vi "get_config_cluster.vi"(8 "error in (no error)":errorcluster, 11 "GenericPlugin in":refnum<class "DetectorYK090623DAQmxAnalog.lvclass">) -> (0 "error out":errorcluster, 2 "config cluster (variant)":variant, 3 "GenericPlugin out":refnum<class "DetectorYK090623DAQmxAnalog.lvclass">)   [LabVIEW 2010, in "DetectorYK090623DAQmxAnalog.lvclass"]
uses:
  DetectorYK090623DAQmxAnalog.lvclass
  DetectorYK090623DAQmxAnalog.lvclass/DetectorYK090623DAQmxAnalog.ctl
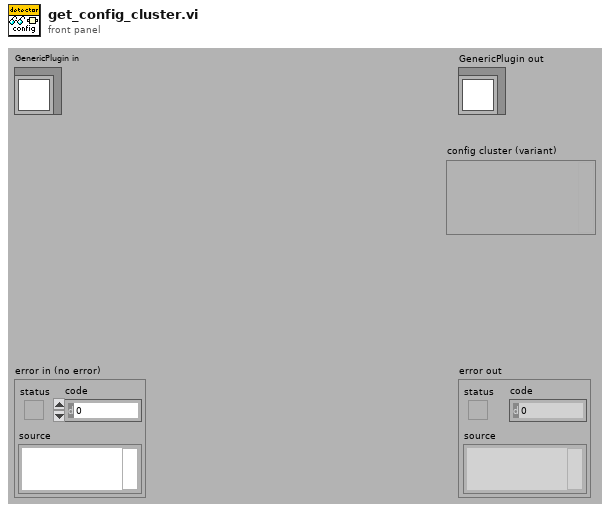
[diagram p1: front panel]
types:
  T1 = typedef "DetectorYK090623DAQmxAnalog.lvclass/config_data_cluster.ctl" = cluster{"manufacturer specification":T2, "type":T3, "LSID":T4, "default voltage":dbl[unit], "analog out":T5}
  T2 = typedef "GenericComponent.lvclass/manufacturer_specification_cluster.ctl" = cluster{"manufacturer":string, "model":string, "serial number":string, "lot number":string}
  T3 = typedef "GenericDetector.lvclass/type_enum.ctl" = enum16{"CCD", "IntensifiedCCD", "AnalogVideo", "PMT", "Photodiode", "Spectoscropy", "LifetimeImaging", "CorrelationSpectroscopy", "FTIR", "EM-CCD", "APD", "CMOS", "Unknown"}
  T4 = typedef "LSID_cluster.ctl" = cluster{"identifier":string, "revision":i32}
  T5 = typedef "plugin_specification.ctl" = cluster{"class path":string, "configuration":string, "label":string, "settings name":string}
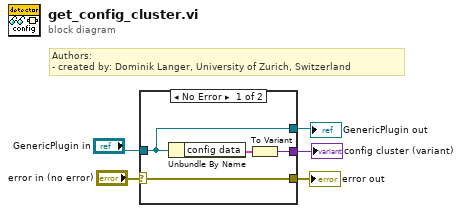
[diagram p0: block diagram]
diagram:
  # "Authors: \n- created by: Dominik Langer, University of Zurich, Switzerland"
  n1 = case shown="No Error" "error in (no error)" {
    selector: "error in (no error)" -> [w7 w11]
    tunnel: "GenericPlugin in" -> [w6 w10]
    tunnel: [w8 _] -> w2
    tunnel: [w7 w11] -> w3
    tunnel: [w6 w10] -> w1
    frame No Error {
      n2 = Unbundle By Name(w6) -> ("config data"=w9:T1)
      n3 = To Variant(anything=w9) -> (Variant=w8:variant)
    }
    frame Error {
    }
  }
  "error out" <- w3
  "GenericPlugin out" <- w1
  "config cluster (variant)" <- w2
